vi "Position Images.vi"(7 "Array of String Ref":refnum<vi>[](array[refnum]), 8 "error in (no error)":errorcluster, 9 "Inspection.Cam Enable-Disable Input":T1, 10 "Image Reference Array":refnum<vi>[](array[refnum]), 11 "ZenGage v3.0 UI.lvclass":refnum<class "ZenGage v3.0 UI.lvclass">) -> (0 "error out":errorcluster)   [LabVIEW 2015]
uses:
  ZenGage v3.0 UI.lvclass
panel:
  in  "Image 1":bool=TRUE
  in  "Image 3":bool=TRUE
  in  "Image 2":bool=TRUE
  out "ZenGage v3.0 UI.lvclass OUT":refnum<class "ZenGage v3.0 UI.lvclass">
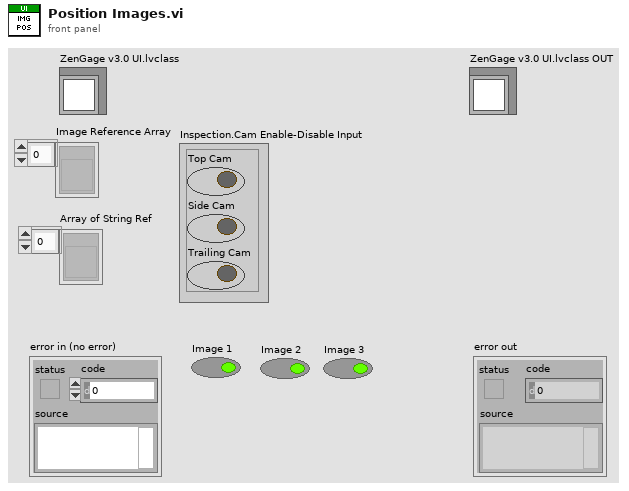
[diagram p1: front panel]
types:
  T1 = cluster{"Top Cam":bool, "Side Cam":bool, "Trailing Cam":bool}
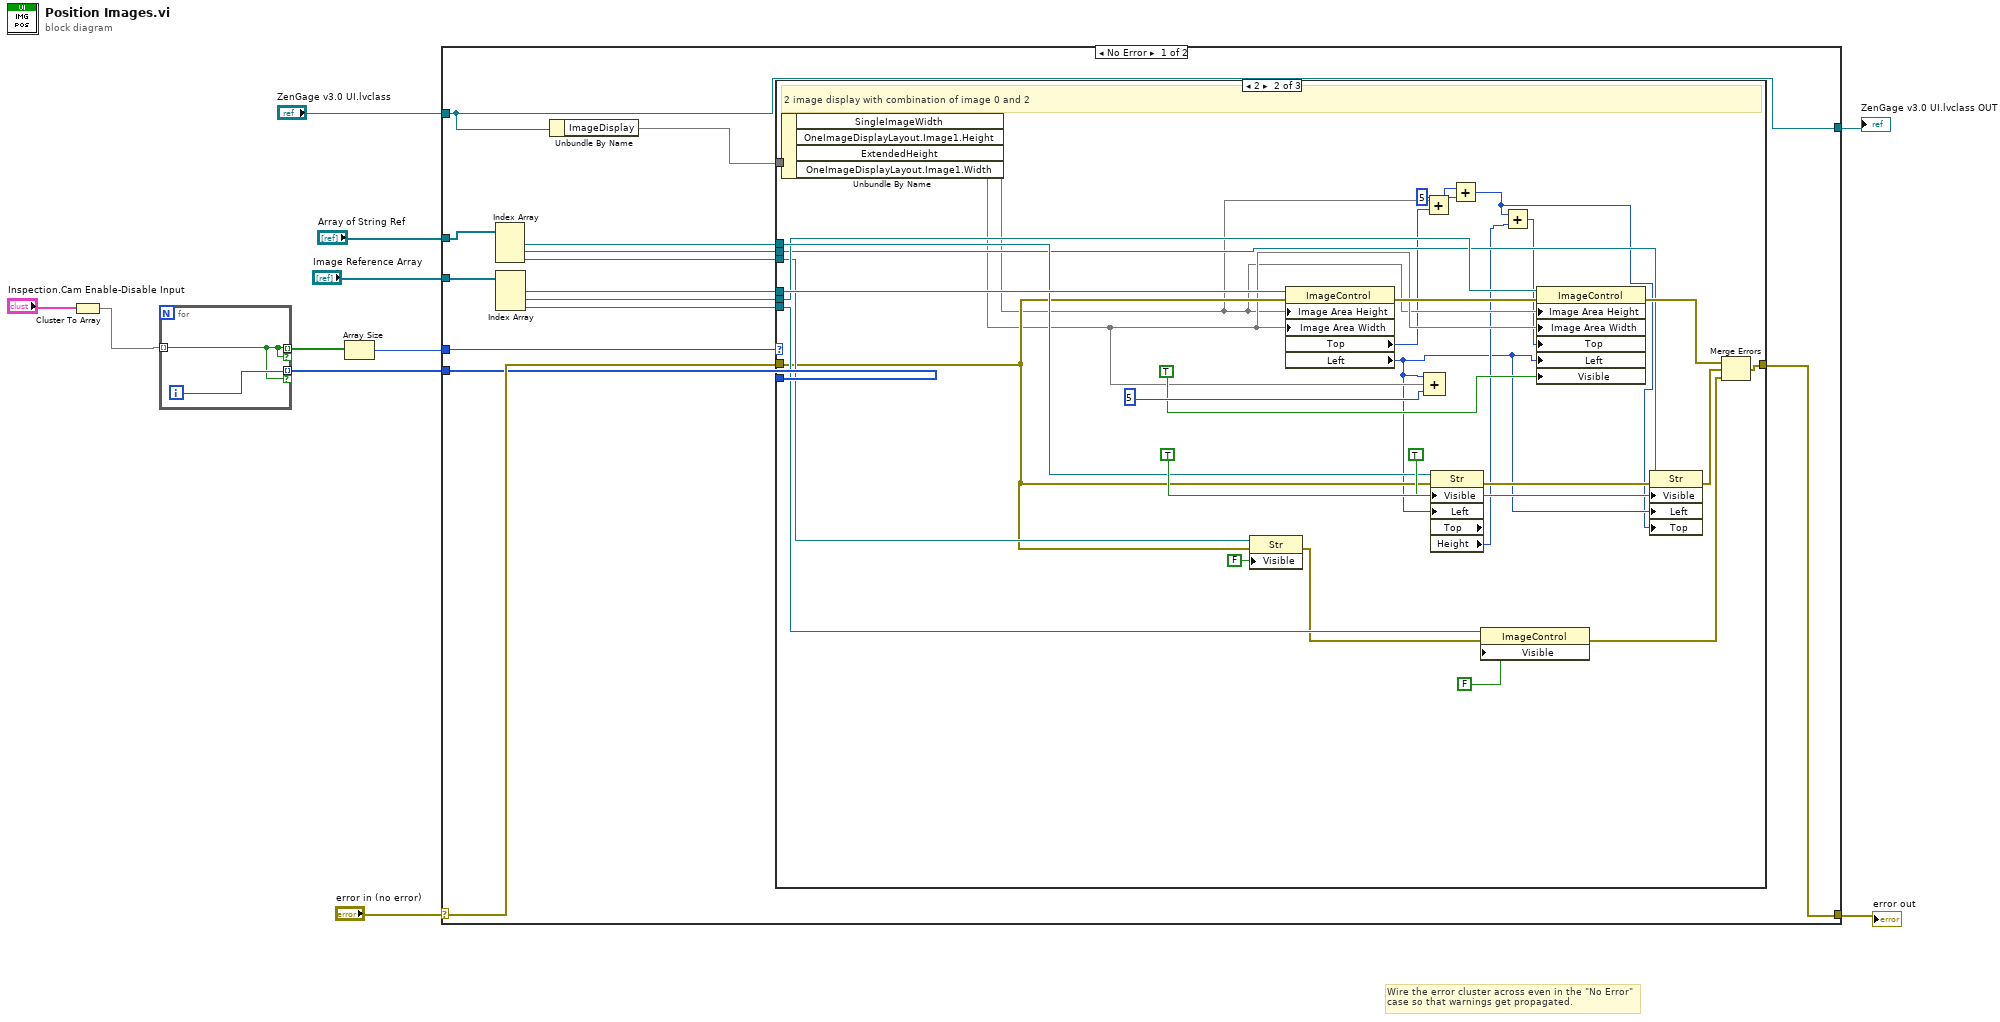
[diagram p0: block diagram]
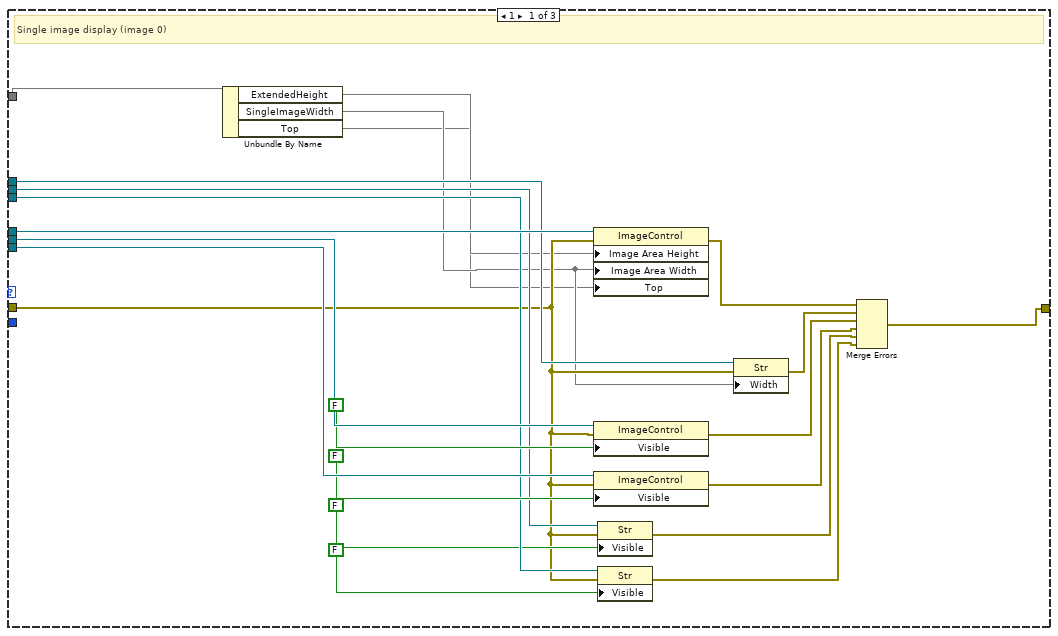
[diagram p2: hidden frame]
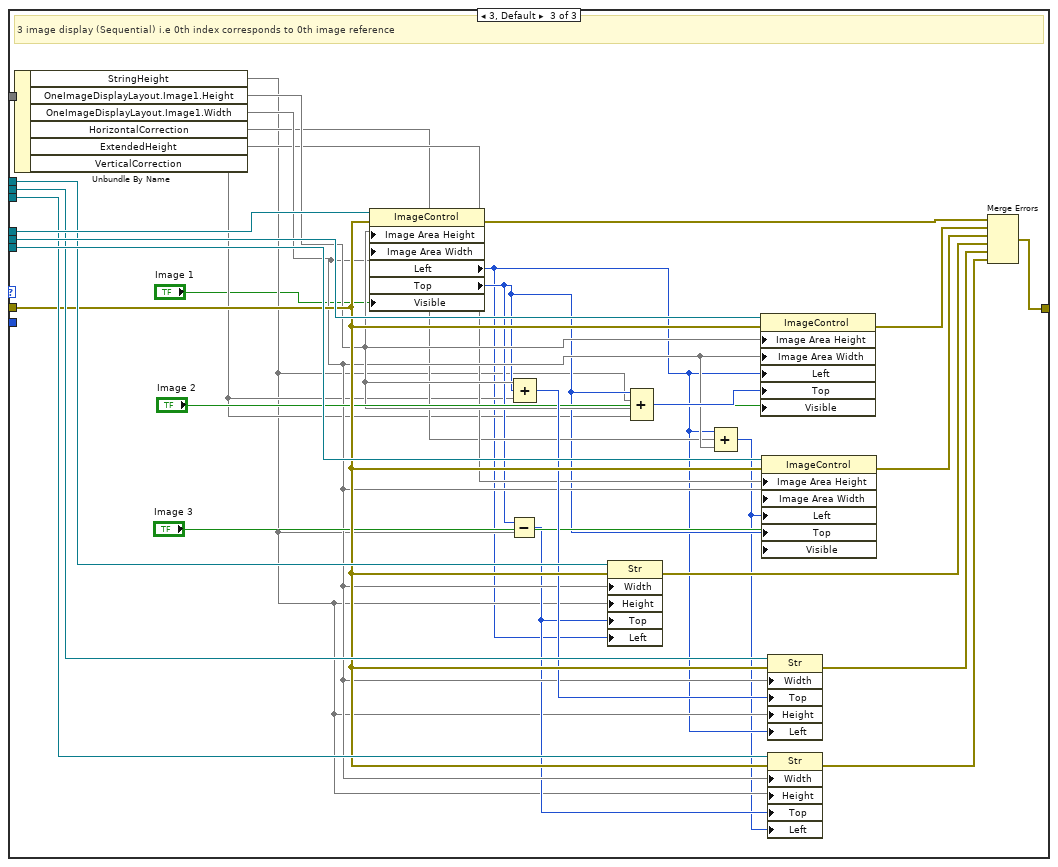
[diagram p3: hidden frame]
diagram:
  # "Wire the error cluster across even in the \"No Error\"\ncase so that warnings get propagated."
  n1 = Cluster To Array(cluster="Inspection.Cam Enable-Disable Input") -> (array=w7:bool[])
  n2 = for {
    tunnel: w7 -> [w12] mode=indexing
    tunnel: [w12] -> w6 mode=indexing if=w12
    tunnel: [w13] -> w3 mode=indexing if=w12
    i -> [w13]
  }
  n3 = Array Size(array=w6) -> (size(s)=w5:i32)
  n4 = case shown="No Error" "error in (no error)" {
    selector: "error in (no error)" -> [w22 w111]
    tunnel: [w21 w111] -> w10
    tunnel: "Image Reference Array" -> [w27 _]
    tunnel: w5 -> [w26 _]
    tunnel: "Array of String Ref" -> [w20 _]
    tunnel: w3 -> [w16 _]
    tunnel: "ZenGage v3.0 UI.lvclass" -> [w15 w110]
    tunnel: [w15 w110] -> w1
    frame No Error {
      n5 = Index Array(array=w20) -> (element #1=w19:refnum<vi>, element #2=w18:refnum<vi>, element #3=w17:refnum<vi>)  [unwired: 3 in]
      n6 = Index Array(array=w27) -> (element #1=w25:refnum<vi>, element #2=w24:refnum<vi>, element #3=w23:refnum<vi>)  [unwired: 3 in]
      n7 = Unbundle By Name(w15) -> ("ImageDisplay"=w14)
      n8 = case shown="2" w26 {
        tunnel: w25 -> [w49 w79 w105]
        tunnel: w24 -> [w44 w67 w104]
        tunnel: w23 -> [w43 w64 w103]
        tunnel: w22 -> [w34 w63 w99]
        tunnel: [w45 w69 w106] -> w21
        tunnel: w19 -> [w48 w73 w102]
        tunnel: w18 -> [w38 w66 w101]
        tunnel: w17 -> [w37 w65 w100]
        tunnel: w16 -> [_ _ _]
        tunnel: w14 -> [w31 w68 w91]
        frame 1 {
          # "Single image display (image 0)"
          n9 = Unbundle By Name(w31) -> ("ExtendedHeight"=w30, "SingleImageWidth"=w29, "Top"=w28)
          n10 = property class="ImageControl"(reference=w49, error in=w34, "Image Area Height"=w30, "Image Area Width"=w29, "Top"=w28) -> (error out=w46:errorcluster)  [unwired: 1 out]
          n11 = property class="ImageControl"(reference=w44, error in=w34, "Visible"=FALSE) -> (error out=w42:errorcluster)  [unwired: 1 out]
          n12 = property class="ImageControl"(reference=w43, error in=w34, "Visible"=FALSE) -> (error out=w41:errorcluster)  [unwired: 1 out]
          n13 = property class="Str"(reference=w38, error in=w34, "Visible"=FALSE) -> (error out=w33:errorcluster)  [unwired: 1 out]
          n14 = property class="Str"(reference=w37, error in=w34, "Visible"=FALSE) -> (error out=w32:errorcluster)  [unwired: 1 out]
          n15 = property class="Str"(reference=w48, error in=w34, "Width"=w29) -> (error out=w47:errorcluster)  [unwired: 1 out]
          n16 = Merge Errors(w46, w47, w42, w41, w33, w32) -> (w45:errorcluster)
        }
        frame 2 {
          # "2 image display with combination of image 0 and 2"
          n17 = Unbundle By Name(w68) -> ("SingleImageWidth"=w58, "OneImageDisplayLayout.Image1.Height"=w57)  [unwired: 2 out]
          n18 = property class="Str"(reference=w65, error in=w63, "Visible"=FALSE) -> (error out=w62:errorcluster)  [unwired: 1 out]
          n19 = property class="ImageControl"(reference=w79, error in=w63, "Image Area Height"=w57, "Image Area Width"=w58) -> (error out=w78:errorcluster, "Top"=w56:i32, "Left"=w53:i32)  [unwired: 1 out]
          n20 = Compound Arithmetic op=ADD(w53, w58, u32 5 ("value")) -> ()  [unwired: 1 out]
          n21 = Add(x=w57, y=w56) -> (x+y=w52:i32)
          n22 = property class="Str" props=["Visible", "Left", "Top", "Height"](reference=w73, error in=w63, "Visible"=TRUE, "Left"=w53) -> (error out=w72:errorcluster, "Height"=w55:u32)  [unwired: 2 out]
          n23 = Add(x=w52, y=5) -> (x+y=w50:i32)
          n24 = property class="ImageControl"(reference=w64, error in=w62, "Visible"=FALSE) -> (error out=w61:errorcluster)  [unwired: 1 out]
          n25 = Add(x=w50, y=w55) -> (x+y=w54:u32)
          n26 = property class="ImageControl"(reference=w67, error in=w78, "Image Area Height"=w57, "Image Area Width"=w58, "Top"=w54, "Left"=w53, "Visible"=TRUE) -> (error out=w70:errorcluster)  [unwired: 1 out]
          n27 = property class="Str"(reference=w66, error in=w72, "Visible"=TRUE, "Left"=w53, "Top"=w50) -> (error out=w71:errorcluster)  [unwired: 1 out]
          n28 = Merge Errors(w70, w71, w61) -> (w69:errorcluster)
        }
        frame 3, Default {
          # "3 image display (Sequential) i.e 0th index corresponds to 0th image reference"
          n29 = Unbundle By Name(w91) -> ("StringHeight"=w83, "OneImageDisplayLayout.Image1.Height"=w90, "OneImageDisplayLayout.Image1.Width"=w89, "HorizontalCorrection"=w86, "ExtendedHeight"=w88, "VerticalCorrection"=w84)
          n30 = property class="ImageControl"(reference=w105, error in=w99, "Image Area Height"=w90, "Image Area Width"=w89, "Visible"="Image 1") -> (error out=w109:errorcluster, "Left"=w82:i32, "Top"=w85:i32)  [unwired: 1 out]
          n31 = Subtract(x=w85, y=w83) -> (x-y=w87:i32)
          n32 = Compound Arithmetic op=ADD(w90, w85, w84) -> (w94:i32)
          n33 = property class="Str"(reference=w102, error in=w99, "Width"=w89, "Height"=w83, "Top"=w87, "Left"=w82) -> (error out=w98:errorcluster)  [unwired: 1 out]
          n34 = Compound Arithmetic op=ADD(w85, w83, w90, w84) -> (w95:i32)
          n35 = Compound Arithmetic op=ADD(w82, w86, w89) -> (w81:i32)
          n36 = property class="ImageControl"(reference=w104, error in=w99, "Image Area Height"=w90, "Image Area Width"=w89, "Left"=w82, "Top"=w95, "Visible"="Image 2") -> (error out=w108:errorcluster)  [unwired: 1 out]
          n37 = property class="ImageControl"(reference=w103, error in=w99, "Image Area Height"=w88, "Image Area Width"=w89, "Left"=w81, "Top"=w85, "Visible"="Image 3") -> (error out=w107:errorcluster)  [unwired: 1 out]
          n38 = property class="Str"(reference=w101, error in=w99, "Width"=w89, "Top"=w94, "Height"=w83, "Left"=w82) -> (error out=w97:errorcluster)  [unwired: 1 out]
          n39 = property class="Str"(reference=w100, error in=w99, "Width"=w89, "Height"=w83, "Top"=w87, "Left"=w81) -> (error out=w96:errorcluster)  [unwired: 1 out]
          n40 = Merge Errors(w109, w108, w107, w98, w97, w96) -> (w106:errorcluster)
        }
      }
    }
    frame Error {
    }
  }
  "error out" <- w10
  "ZenGage v3.0 UI.lvclass OUT" <- w1
